vi "Cluster Sample.vi"() -> ()   [LabVIEW 2025]
panel:
  out "Student 2":T1
  out "Student":T1
  in  "student name":string
  in  "Cgpa":dbl
  in  "student email":string
  in  "student mobile":dbl
  in  "student age":dbl
  out "?":string
  out "?":string
  out "?":string
  out "Name unbundled by name":string
  out "age unbundleby name":dbl
  out "Company name":string
  out "Physically Disabled?":bool
  out "Gender":enum16{"", "Male\n", "Female\n"}(ring)
  out "Name":string
  out "Age":dbl
  in  "Employee":T2
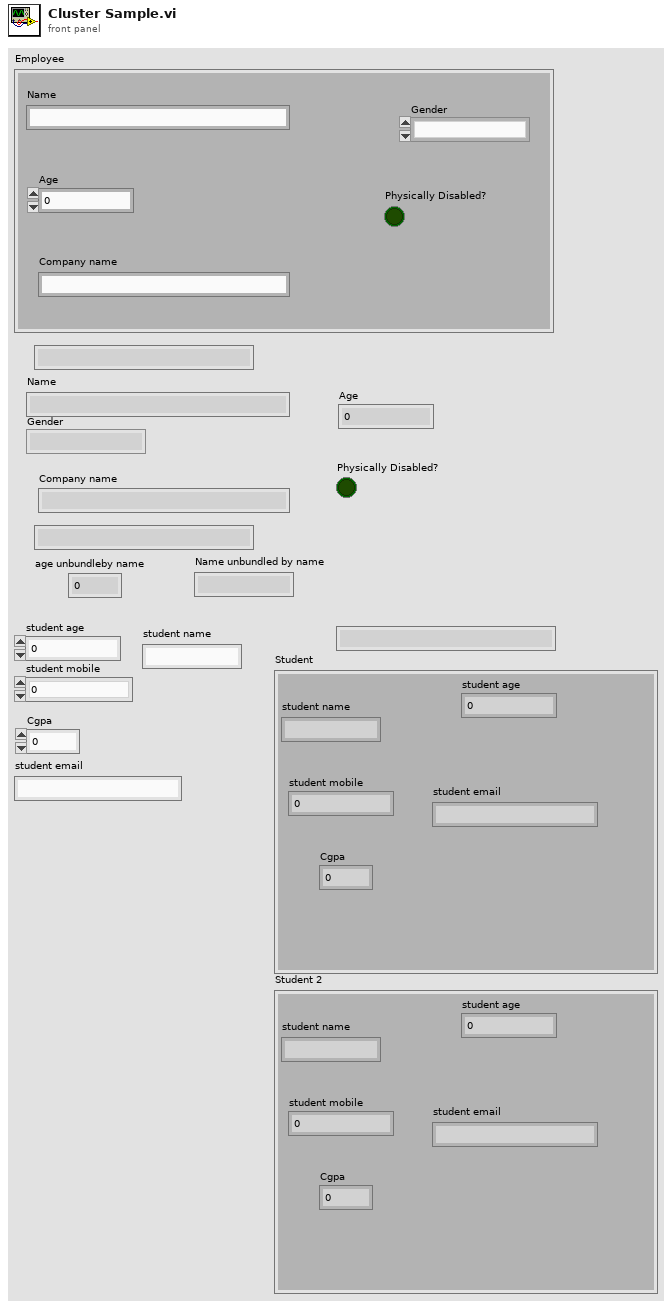
[diagram p1: front panel]
types:
  T1 = cluster{"student name":string, "student age":dbl, "student mobile":dbl, "student email":string, "Cgpa":dbl}
  T2 = cluster{"Age":dbl, "Name":string, "Gender":enum16{"", "Male\n", "Female\n"}, "Physically Disabled?":bool, "Company name":string}
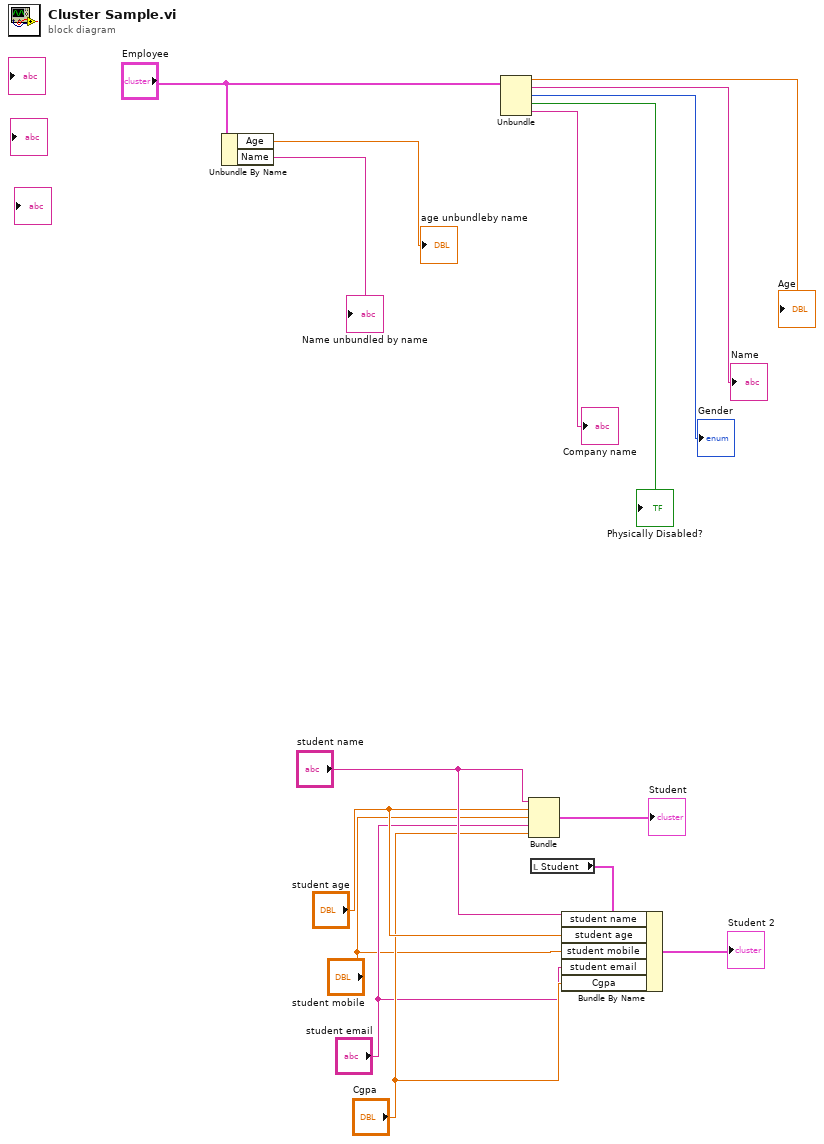
[diagram p0: block diagram]
diagram:
  n1 = Unbundle By Name("Employee") -> ("Age"=→"age unbundleby name":dbl, "Name"=→"Name unbundled by name":string)
  n2 = Unbundle("Employee") -> ("Age"=→"Age":dbl, "Name"=→"Name":string, "Gender"=→"Gender":enum16{"", "Male\n", "Female\n"}, "Physically Disabled?"=→"Physically Disabled?":bool, "Company name"=→"Company name":string)
  n3 = Bundle("student name"="student name", "student age"="student age", "student mobile"="student mobile", "student email"="student email", "Cgpa"="Cgpa") -> (→"Student":T1)  [unwired: 1 in]
  n4 = local read "Student"() -> (w7:T1)
  n5 = Bundle By Name(cluster=w7, "student name"="student name", "student age"="student age", "student mobile"="student mobile", "student email"="student email", "Cgpa"="Cgpa") -> (→"Student 2":T1)
